vi "Button press.vi"(0 "Up":bool, 5 "Down":bool, 7 "Left":bool, 9 "Right":bool, 11 "Stop":bool) -> (4 "Command":T1(ring), 6 "angle":dbl)   [LabVIEW 2017]
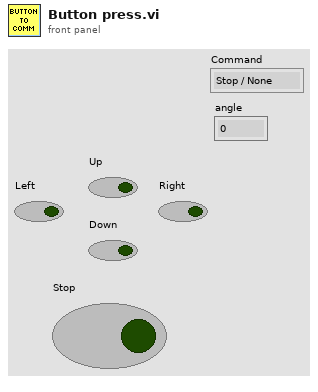
[diagram p1: front panel]
types:
  T1 = enum16{"Stop / None", "Forward", "Backward", "Left", "Right", "Manual"}
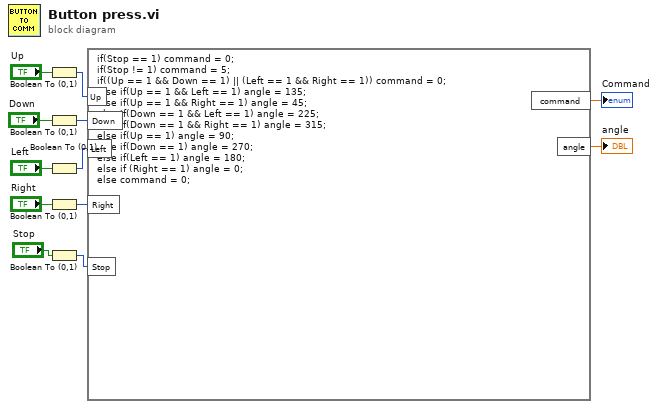
[diagram p0: block diagram]
diagram:
  n1 = Boolean To (0,1)(Boolean="Up") -> (0, 1=w11:i16)
  n2 = Boolean To (0,1)(Boolean="Down") -> (0, 1=w9:i16)
  n3 = Boolean To (0,1)(Boolean="Left") -> (0, 1=w7:i16)
  n4 = Boolean To (0,1)(Boolean="Right") -> (0, 1=w5:i16)
  n5 = Boolean To (0,1)(Boolean="Stop") -> (0, 1=w1:i16)
  n6 = formula code="if(Stop == 1) command = 0;\nif(Stop != 1) command = 5;\nif((Up == 1 && Down == 1) || (Left == 1 && Right == 1)) command = 0;\nelse if(Up == 1 && Left == 1) angle = 135;\nelse if(Up == 1 && Right == 1) angle = 45;\nelse if(Down == 1 && Left == 1) angle = 225;\nelse if(Down == 1 && Right == 1) angle = 315;\nelse if(Up == 1) angle = 90;\nelse if(Down == 1) angle = 270;\nelse if(Left == 1) angle = 180;\nelse if (Right == 1) angle = 0;\nelse command = 0;"("Up"=w11, "Down"=w9, "Left"=w7, "Right"=w5, "Stop"=w1) -> ("command"=→"Command":dbl, "angle"=→"angle":dbl)
